vi "Create FP Item.vi"(6 "Cluster Component":bool, 8 "error in (no error)":errorcluster, 10 "GObject In":refnum<vi>, 11 "GProgressbar in":refnum<class "Progressbar.lvclass">) -> (0 "error out":errorcluster, 1 "Is Control":bool, 2 "Is Indicator":bool, 3 "GProgressbar out":refnum<class "Progressbar.lvclass">, 4 "All Objects Created":refnum<class "Object.lvclass">[](array[class]), 5 "Is Visible":bool)   [LabVIEW 2017, in "Front Panel Publisher.lvlib" / "Progressbar.lvclass"]
uses:
  Progressbar.lvclass
  Control_class/Control.lvclass
  Object_class/Object.lvclass
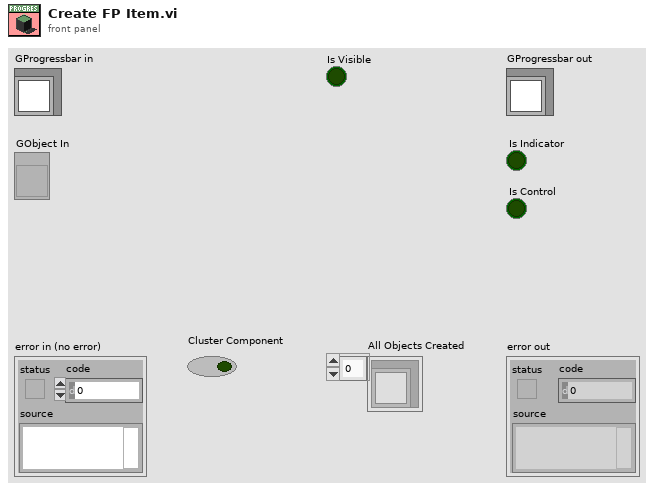
[diagram p1: front panel]
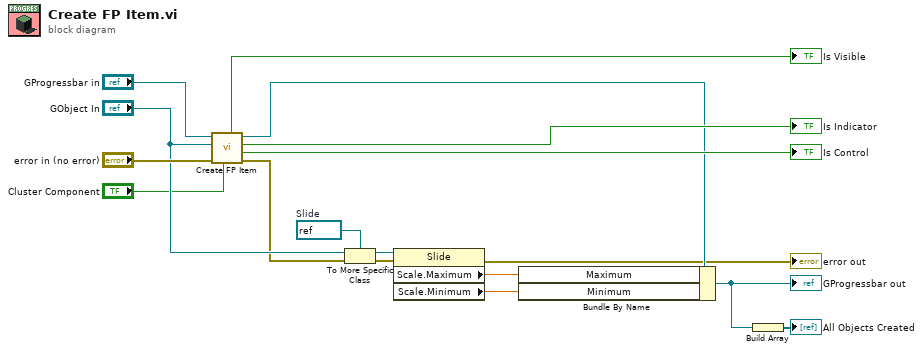
[diagram p0: block diagram]
diagram:
  w11 = refnum<vi> refnum  # Slide
  n1 = call-parent "Create FP Item.vi"("Cluster Component"="Cluster Component", "error in (no error)"="error in (no error)", "GObject In"="GObject In", "GControl in"="GProgressbar in") -> ("error out"=w5:errorcluster, "Is Control"=→"Is Control":bool, "Is Indicator"=→"Is Indicator":bool, "GControl out"=w15:refnum<class "Progressbar.lvclass">, "Is Visible"=→"Is Visible":bool)  [unwired: 2 in, 1 out]
  n2 = To More Specific Class(target class=w11, reference="GObject In", error in=w5) -> (specific class reference=w9:refnum<vi>, error out=w10:errorcluster)
  n3 = property class="Slide"(reference=w9, error in=w10) -> (error out=→"error out":errorcluster, "Scale.Maximum"=w7:dbl, "Scale.Minimum"=w6:dbl)  [unwired: 1 out]
  n4 = Bundle By Name(cluster=w15, "Maximum"=w7, "Minimum"=w6) -> (w3:refnum<class "Progressbar.lvclass">)
  "GProgressbar out" <- w3
  n5 = Build Array(w3) -> (→"All Objects Created":refnum<class "Progressbar.lvclass">[])
